vi "Erase Device.vi"(8 "error in (no error)":errorcluster, 11 "MPLab in":refnum<class "MPLab.lvclass">) -> (0 "error out":errorcluster, 3 "MPLab out":refnum<class "MPLab.lvclass">)   [LabVIEW 2018, in "MPLab.lvlib" / "MPLab.lvclass"]
uses:
  MPLab.lvclass
  Custom Controls/Command Line Options.ctl
  MPLab.lvclass/MPLab.ctl
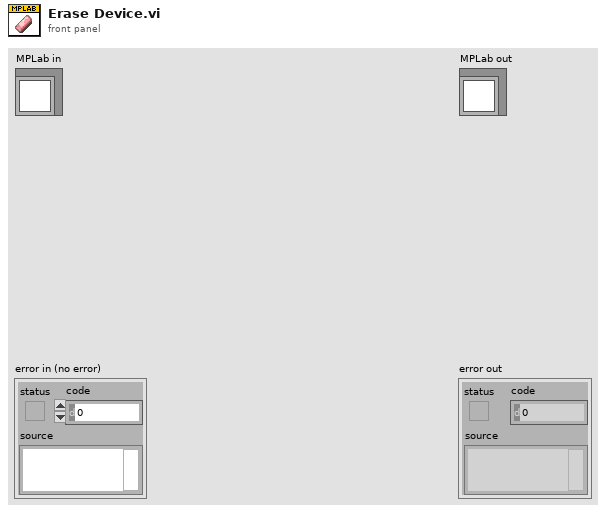
[diagram p1: front panel]
types:
  T1 = typedef "MPLab.lvlib/MPLab.lvclass/Command Line Options.ctl" = enum16{"Blank Check Device", "Erase Flash Device", "Hex File", "Display Device ID", "Display File Checksum", "Low Voltage Programming", "Memory Region", "Part", "Tool", "Verify Device"}
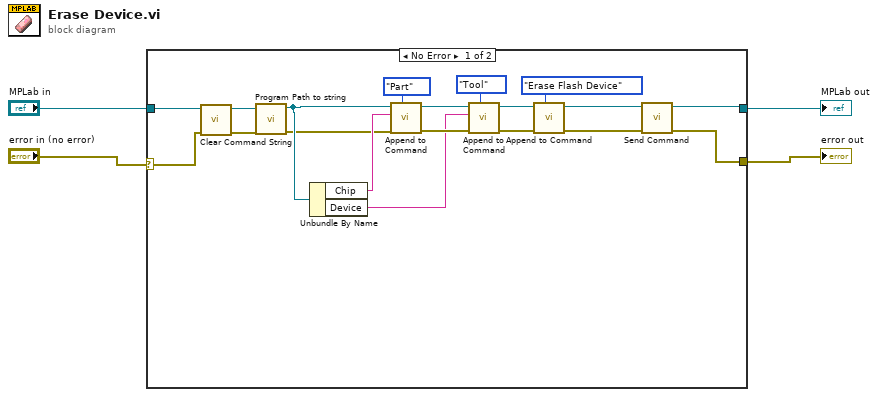
[diagram p0: block diagram]
diagram:
  n1 = case shown="No Error" "error in (no error)" {
    selector: "error in (no error)" -> [w22 w25]
    tunnel: [w5 w25] -> w2
    tunnel: [w7 w24] -> w3
    tunnel: "MPLab in" -> [w23 w24]
    frame No Error {
      n2 = call "Clear Command String.vi"("error in (no error)"=w22, "MPLab in"=w23) -> ("error out"=w21:errorcluster, "MPLab out"=w20:refnum<class "MPLab.lvclass">)  [unwired: 8 in]
      n3 = call "Program Path to string.vi"("error in"=w21, "MPLab in"=w20) -> ("error out"=w16:errorcluster, "MPLab out"=w17:refnum<class "MPLab.lvclass">)  [unwired: 8 in]
      n4 = Unbundle By Name(w17) -> ("Chip"=w19:string, "Device"=w13:string)
      n5 = call "Append to Command.vi"("Command Line Options"=Command_Line_Options."Part", "error in (no error)"=w16, "Parameter"=w19, "MPLab in"=w17) -> ("error out"=w15:errorcluster, "MPLab out"=w14:refnum<class "MPLab.lvclass">)  [unwired: 6 in]
      n6 = call "Append to Command.vi"("Command Line Options"=Command_Line_Options."Tool", "error in (no error)"=w15, "Parameter"=w13, "MPLab in"=w14) -> ("error out"=w11:errorcluster, "MPLab out"=w10:refnum<class "MPLab.lvclass">)  [unwired: 6 in]
      n7 = call "Append to Command.vi"("Command Line Options"=Command_Line_Options."Erase Flash Device", "error in (no error)"=w11, "MPLab in"=w10) -> ("error out"=w6:errorcluster, "MPLab out"=w8:refnum<class "MPLab.lvclass">)  [unwired: 7 in]
      n8 = call "Send Command.vi"("error in"=w6, "MPLab in"=w8) -> ("error out"=w5:errorcluster, "MPLab out"=w7:refnum<class "MPLab.lvclass">)  [unwired: 8 in]
    }
    frame Error {
    }
  }
  "error out" <- w2
  "MPLab out" <- w3
